vi "Main.vi"(10 "Coins Panel":refnum<vi>, 11 "Module Admin":refnum<class "Delacor_lib_QMH_Module Admin.lvclass">) -> ()   [LabVIEW 2019, in "COINS.lvlib"]
doc: "This template is based off of the Queued Message Handler design pattern and the Queued Message Handler project template that ships with LabVIEW.\n\nThe main difference is that the queue is private to this module and communication between modules is performed via Broadcast and Request events.\n\nRequest events are wrapped in public API methods and are handled in the Event Handling Loop (EHL) of this VI. Any module can register for Broadcast events sent by this module. The EHL generates messages based on user interface actions.\n\nThe Message Handling Loop (MHL) processes messages generated by the EHL, or by other messages. The messages are string values, so new messages can be added easily to the Message Cases case structure in the MHL. Each message cluster can also provide an optional value for Message Data, which is a variant that can be converted to whatever message-specific data is required.\n_____\nBased on Delacor QMH Project Template 5.0.0.82."
uses:
  COINS.lvlib
  <vilib>/Delacor/Delacor QMH/Libraries/Module Admin_class/Delacor_lib_QMH_Module Admin.lvclass
  Module Data--cluster.ctl
  Stop Argument--cluster.ctl
  <vilib>/Delacor/Delacor QMH/Libraries/Message Queue_class/Delacor_lib_QMH_Message Queue.lvclass/Delacor_lib_QMH_Message Queue.ctl
  <vilib>/Delacor/Delacor QMH/Libraries/Module Admin_class/Delacor_lib_QMH_Module Admin.lvclass/Delacor_lib_QMH_Module Admin.ctl
  SET COINS Argument--cluster.ctl
  UPDATE COIN Argument--cluster.ctl
  UPDATE CREDIT Argument--cluster.ctl
  <vilib>/Delacor/Delacor QMH/Libraries/Message Queue_class/Delacor_lib_QMH_Enqueue Message (Single).vi
  <vilib>/Delacor/Delacor QMH/Libraries/Module Admin_class/Delacor_lib_QMH_Get External Launch.vi
  <vilib>/Utility/error.llb/Error Cluster From Error Code.vi
  <vilib>/ErrorRing/Error Ring.xnode
  <vilib>/Delacor/Delacor QMH/Libraries/Message Queue_class/Delacor_lib_QMH_Message Queue.lvclass
  MESSAGES/MESSAGES.lvlib
panel:
  in  "COIN 1":bool
  in  "COIN 2":bool
  in  "COIN 3":bool
  in  "COIN 4":bool
  out "error out":errorcluster
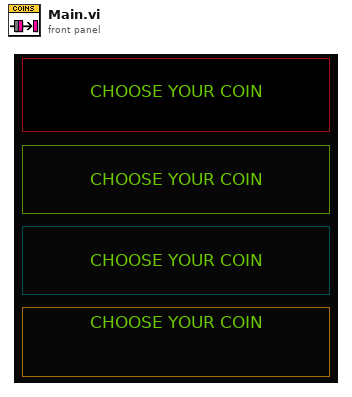
[diagram p1: front panel]
types:
  T1 = typedef "COINS.lvlib/Request Events--cluster.ctl" = cluster{"Stop Module":refnum<user-event>, "Show Panel":refnum<user-event>, "Hide Panel":refnum<user-event>, "Get Module Execution Status":refnum<user-event>, "Show Diagram":refnum<user-event>, "SET COINS":refnum<user-event>, "UPDATE COIN":refnum<user-event>, "UPDATE CREDIT":refnum<user-event>}
  T2 = typedef "COINS.lvlib/Module Data--cluster.ctl" = cluster{"Status":string, "CREDIT":dbl, "PRICE":dbl, "CHANGE":dbl, "MONEY COINS":string[], "MONEY VALUES":string[], "COINS":bool[]}
  T3 = enum32{"invalid lock state", "Not Locked", "Locked (No Password)", "Password-protected"}
  T4 = typedef "COINS.lvlib/Stop Argument--cluster.ctl" = cluster{"Origin":string, "Exit via Stop Module Req?":bool, "Wait for Module to stop?":bool}
  T5 = typedef "COINS.lvlib/SET COINS Argument--cluster.ctl" = cluster{"MONEY ARRAY":string[]}
  T6 = typedef "COINS.lvlib/UPDATE COIN Argument--cluster.ctl" = cluster{"Boolean":bool}
  T7 = typedef "COINS.lvlib/UPDATE CREDIT Argument--cluster.ctl" = cluster{"Boolean":bool}
  T8 = enum32{"Invalid", "Standard", "Closed", "Hidden", "Minimized", "Maximized"}
  T9 = cluster{"MONEY ARRAY[0]":string, "MONEY ARRAY[1]":string, "MONEY ARRAY[2]":string, "MONEY ARRAY[3]":string, "MONEY ARRAY[4]":string, "MONEY ARRAY[5]":string, "MONEY ARRAY[6]":string, "MONEY ARRAY[7]":string, "MONEY ARRAY[8]":string}
  T10 = cluster{"MONEY COINS[0]":string, "MONEY COINS[1]":string, "MONEY COINS[2]":string, "MONEY COINS[3]":string, "MONEY COINS[4]":string, "MONEY COINS[5]":string, "MONEY COINS[6]":string, "MONEY COINS[7]":string, "MONEY COINS[8]":string}
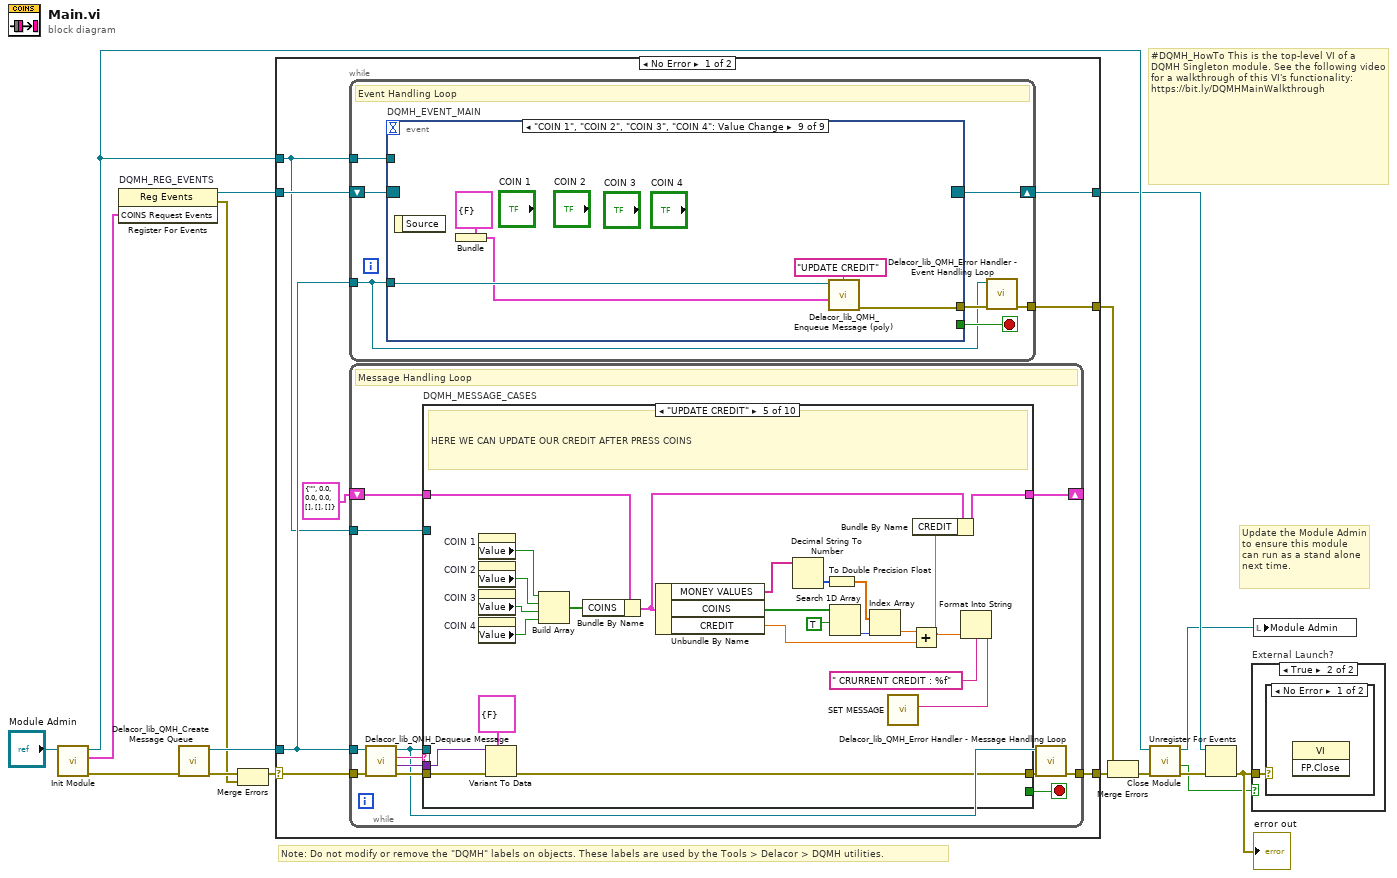
[diagram p0: block diagram]
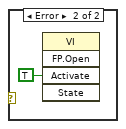
[diagram p3: hidden frame]
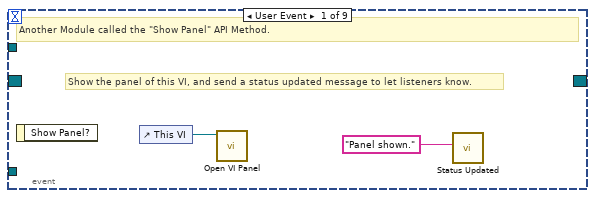
[diagram p4: hidden frame]
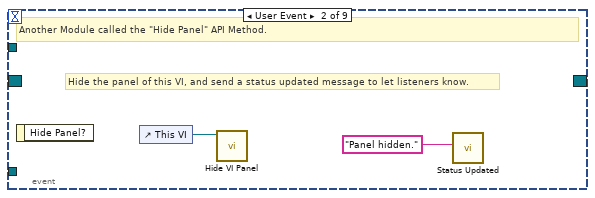
[diagram p5: hidden frame]
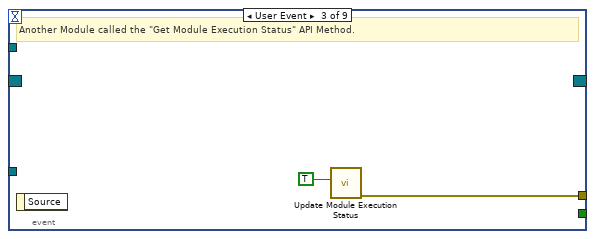
[diagram p6: hidden frame]
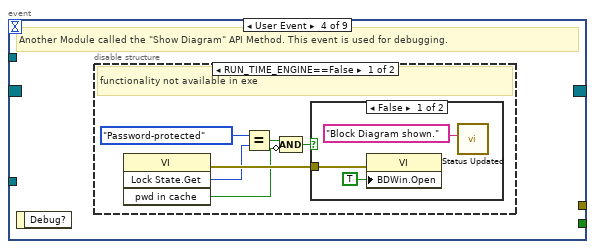
[diagram p7: hidden frame]
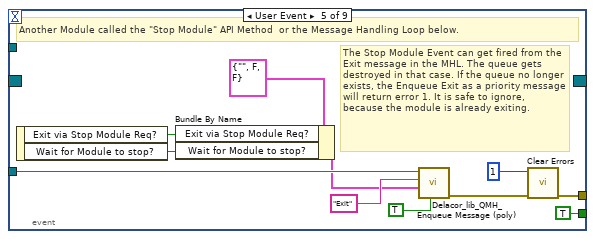
[diagram p10: hidden frame]
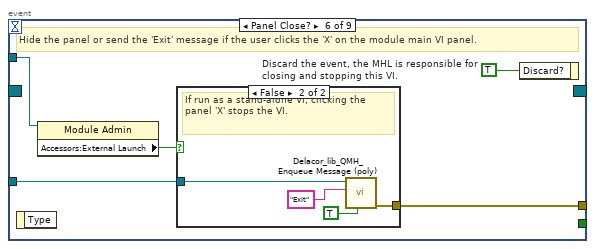
[diagram p11: hidden frame]
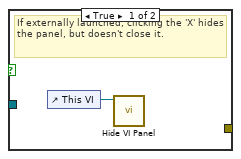
[diagram p12: hidden frame]
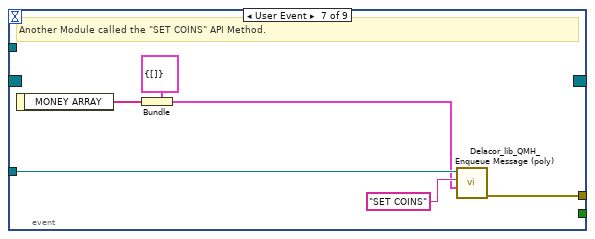
[diagram p13: hidden frame]
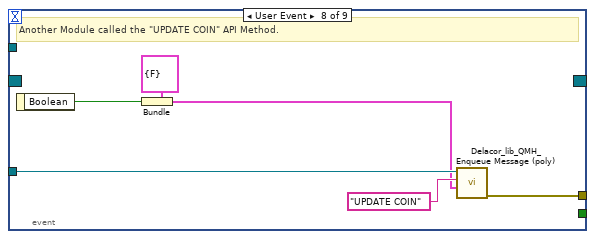
[diagram p14: hidden frame]
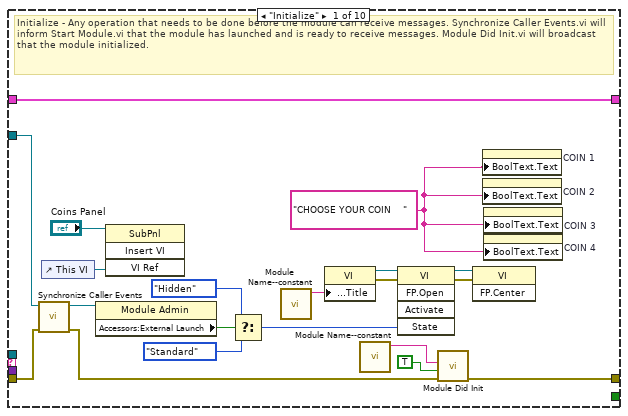
[diagram p15: hidden frame]
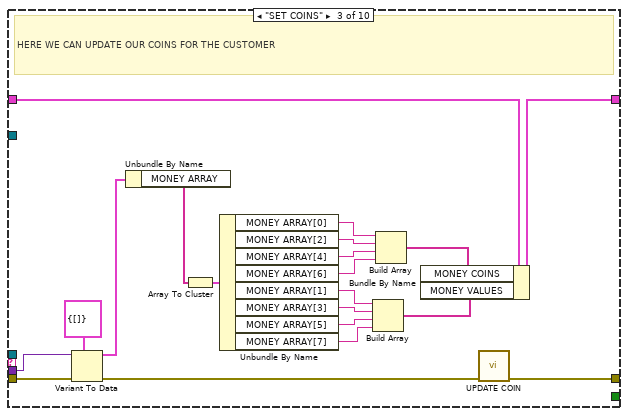
[diagram p17: hidden frame]
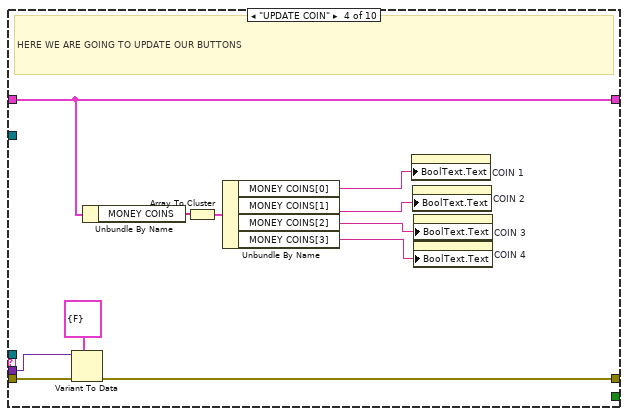
[diagram p18: hidden frame]
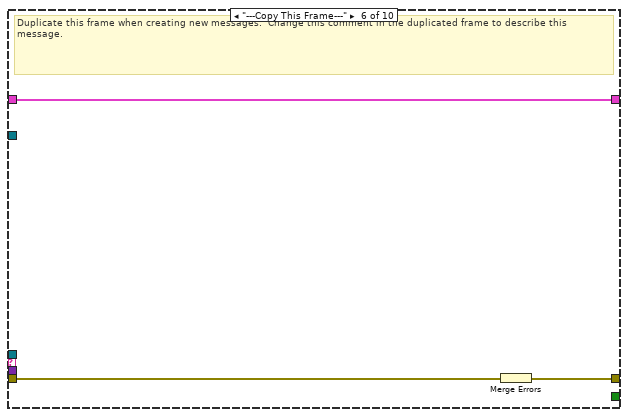
[diagram p19: hidden frame]
diagram:
  # "#DQMH_HowTo This is the top-level VI of a DQMH Singleton module. See the following video for a walkthrough of this VI's functionality: https://bit.ly/DQMHMainWalkthrough"
  # "Note: Do not modify or remove the \"DQMH\" labels on objects. These labels are used by the Tools > Delacor > DQMH utilities."
  # "Update the Module Admin to ensure this module can run as a stand alone next time."
  n1 = call "Init Module.vi"("Singleton Module Admin in"="Module Admin") -> ("error out"=w16:errorcluster, "COINS Request Events"=w6:T1, "Singleton Module Admin out"=w9:refnum<class "Delacor_lib_QMH_Module Admin.lvclass">)  [unwired: 8 in]
  n2 = register-events "DQMH_REG_EVENTS"(w6) -> (reference out=w7:refnum<event-registration>, error out=w1:errorcluster)  [unwired: 2 in]
  n3 = call <vilib>:"Delacor_lib_QMH_Create Message Queue.vi"("error in (no error)"=w16) -> ("error out"=w11:errorcluster, "Message Queue"=w5:refnum<class "Delacor_lib_QMH_Message Queue.lvclass">)  [unwired: 9 in]
  n4 = Merge Errors(w11, w1) -> (w10:errorcluster)
  n5 = case shown="No Error" w10 {
    selector: w10 -> [w23 w227]
    tunnel: [w25 w226] -> w17
    tunnel: [w22 w232] -> w8
    tunnel: w7 -> [w20 w232]
    tunnel: w5 -> [w19 w225]
    tunnel: [w24 _] -> w14
    tunnel: w9 -> [w18 w228]
    frame No Error {
      n6 = while {
        tunnel: w19 -> [w26]
        shift-right: [w29] -> w22
        shift-left: w20 -> [w30]
        tunnel: [w31] -> w24
        tunnel: w18 -> [w27]
        stop <- w28 stop-if-true
        # "Event Handling Loop"
        n7 = event "DQMH_EVENT_MAIN" shown="[8] \"COIN 1\", \"COIN 2\", \"COIN 3\", \"COIN 4\": Value Change" {
          selector: w30 -> [_ _ _ _ _ _ _ _ _]
          dyn-events: [_ _ _ _ _ _ _ _ _] -> w29
          timeout: _ -> [_ _ _ _ _ _ _ _ _]
          tunnel: [_ _ _ _ TRUE ("Discard?") _ _ _ _] -> w28
          tunnel: w26 -> [_ _ _ _ w54 w61 w74 w80 w83]
          tunnel: [_ _ w38 _ w57 w63 w69 w75 w84] -> w32
          tunnel: w27 -> [_ _ _ _ _ w60 _ _ _]
          event User Event {
            # "Show the panel of this VI, and send a status updated message to let listeners know."
            # "Another Module called the \"Show Panel\" API Method."
            n8 = event-data() -> ()  [unwired: 1 in, 1 out]
            n9 = control-ref of="This VI"() -> (w34:refnum<vi>)
            n10 = call "Open VI Panel.vi"("VI"=w34) -> ()  [unwired: 10 in, 1 out]
            n11 = call "Status Updated.vi"("Status"="Panel shown." ("format string")) -> ()  [unwired: 10 in, 1 out]
          }
          event User Event {
            # "Hide the panel of this VI, and send a status updated message to let listeners know."
            # "Another Module called the \"Hide Panel\" API Method."
            n12 = event-data() -> ()  [unwired: 1 in, 1 out]
            n13 = control-ref of="This VI"() -> (w36:refnum<vi>)
            n14 = call "Hide VI Panel.vi"("VI"=w36) -> ()  [unwired: 10 in, 1 out]
            n15 = call "Status Updated.vi"("Status"="Panel hidden." ("format string")) -> ()  [unwired: 10 in, 1 out]
          }
          event User Event {
            # "Another Module called the \"Get Module Execution Status\" API Method."
            n16 = event-data() -> ()  [unwired: 1 in, 1 out]
            n17 = call "Update Module Execution Status.vi"("Running?"=TRUE) -> ("error out"=w38:errorcluster)  [unwired: 10 in]
          }
          event User Event {
            # "Another Module called the \"Show Diagram\" API Method. This event is used for debugging."
            n18 = event-data() -> ()  [unwired: 1 in, 1 out]
            n19 = disable-structure shown="RUN_TIME_ENGINE==False" {
              frame condition #0 (active) {
                # "functionality not available in exe"
                n20 = invoke class="VI" method="Lock State.Get"() -> (error out=w44:errorcluster, "Get Lock State"=w43:T3, "pwd in cache"=w40:bool)  [unwired: 4 in, 1 out]
                n21 = Equal?(x=T3."Password-protected", y=w43) -> (x = y?=w41:bool)
                n22 = Compound Arithmetic op=AND(w41, invert w40) -> (w39:bool)
                n23 = case shown="False" w39 {
                  tunnel: w44 -> [w47 _]
                  frame False {
                    n24 = property class="VI"(error in=w47, "BDWin.Open"=TRUE ("Block Diagram Window:Open")) -> ()  [unwired: 1 in, 2 out]
                    n25 = call "Status Updated.vi"("Status"="Block Diagram shown." ("format string")) -> ()  [unwired: 10 in, 1 out]
                  }
                  frame True {
                    # "Password-protected VI, and the password is not in the cache. Do not show the diagram."
                  }
                }
              }
              frame condition #1 {
              }
            }
          }
          event User Event {
            # "The Stop Module Event can get fired from the Exit message in the MHL. The queue gets destroyed in that case. If the queue no longer exists, the Enqueue Exit as a priority message will return error 1. It is safe to ignore, because the module is already exiting."
            # "Another Module called the \"Stop Module\" API Method  or the Message Handling Loop below."
            n26 = event-data() -> ("Exit via Stop Module Req?"=w50:bool, "Wait for Module to stop?"=w49:bool)  [unwired: 1 in]
            n27 = Bundle By Name(cluster=T4 {"Origin"="", "Exit via Stop Module Req?"=FALSE, "Wait for Module to stop?"=FALSE} ("Stop Argument"), "Exit via Stop Module Req?"=w50, "Wait for Module to stop?"=w49) -> (w48:T4)
            n28 = call-poly <vilib>:"Delacor_lib_QMH_Enqueue Message (poly).vi"("Priority Message? (F)"=TRUE, "Message Data"=w48, "Message"="Exit", "Message Queue in"=w54) -> ("error out"=w58:errorcluster)  [unwired: 6 in, 1 out]
            n29 = call <vilib>:"Clear Errors.vi"("error in (no error)"=w58, "specific error code to clear (0: all)"=1) -> ("error out"=w57:errorcluster)  [unwired: 4 in, 1 out]
          }
          event Panel Close? {
            w62 = TRUE  # Discard the event, the MHL is responsible for closing and stopping this VI.
            # "Hide the panel or send the 'Exit' message if the user clicks the 'X' on the module main VI panel."
            n30 = event-data() -> ()  [unwired: 1 in, 1 out]
            n31 = property class="Module Admin"(reference=w60) -> ("Accessors:External Launch"=w59:bool)  [unwired: 1 in, 2 out]
            n32 = case shown="False" w59 {
              tunnel: w61 -> [_ w67]
              tunnel: [_ w68] -> w63
              frame True {
                # "If externally launched, clicking the 'X' hides the panel, but doesn't close it."
                n33 = control-ref of="This VI"() -> (w64:refnum<vi>)
                n34 = call "Hide VI Panel.vi"("VI"=w64) -> ()  [unwired: 10 in, 1 out]
              }
              frame False {
                # "If run as a stand-alone VI, clicking the panel 'X' stops the VI."
                n35 = call-poly <vilib>:"Delacor_lib_QMH_Enqueue Message (poly).vi"("Priority Message? (F)"=TRUE, "Message"="Exit", "Message Queue in"=w67) -> ("error out"=w68:errorcluster)  [unwired: 7 in, 1 out]
              }
            }
            n36 = event-data("Discard?"=w62) -> ()  [unwired: 1 in, 1 out]
          }
          event User Event {
            # "Another Module called the \"SET COINS\" API Method."
            n37 = event-data() -> ("MONEY ARRAY"=w70:string[])  [unwired: 1 in]
            n38 = Bundle(cluster=T5 {"MONEY ARRAY"=[]} ("SET COINS Argument"), "MONEY ARRAY"=w70) -> (w71:T5)
            n39 = call-poly <vilib>:"Delacor_lib_QMH_Enqueue Message (poly).vi"("Message Data"=w71, "Message"="SET COINS", "Message Queue in"=w74) -> ("error out"=w69:errorcluster)  [unwired: 7 in, 1 out]
          }
          event User Event {
            # "Another Module called the \"UPDATE COIN\" API Method."
            n40 = event-data() -> ("Boolean"=w76:bool)  [unwired: 1 in]
            n41 = Bundle(cluster=T6 {"Boolean"=FALSE} ("UPDATE COIN Argument"), "Boolean"=w76) -> (w77:T6)
            n42 = call-poly <vilib>:"Delacor_lib_QMH_Enqueue Message (poly).vi"("Message Data"=w77, "Message"="UPDATE COIN", "Message Queue in"=w80) -> ("error out"=w75:errorcluster)  [unwired: 7 in, 1 out]
          }
          event "COIN 1", "COIN 2", "COIN 3", "COIN 4": Value Change {
            n43 = event-data() -> ()  [unwired: 1 in, 1 out]
            n44 = Bundle(cluster=T7 {"Boolean"=FALSE} ("UPDATE CREDIT Argument")) -> (w81:T7)  [unwired: 1 in]
            n45 = call-poly <vilib>:"Delacor_lib_QMH_Enqueue Message (poly).vi"("Message Data"=w81, "Message"="UPDATE CREDIT", "Message Queue in"=w83) -> ("error out"=w84:errorcluster)  [unwired: 7 in, 1 out]
          }
        }
        n46 = call-dynamic "Delacor_lib_QMH_Error Handler - Event Handling Loop.vi"("error in (no error)"=w32, "Message Queue in"=w26) -> ("dup error in"=w31:errorcluster)  [unwired: 8 in, 1 out]
      }
      n47 = while {
        tunnel: w19 -> [w88]
        shift-right: [w92] -> _
        shift-left: T2 {"Status"="", "CREDIT"=0.0, "PRICE"=0.0, "CHANGE"=0.0, "MONEY COINS"=[], "MONEY VALUES"=[], "COINS"=[]} ("Data Cluster") -> [w93]
        tunnel: w23 -> [w96]
        tunnel: [w94] -> w25
        tunnel: w18 -> [w86]
        stop <- w91 stop-if-true
        # "Message Handling Loop"
        n48 = call-dynamic "Delacor_lib_QMH_Dequeue Message.vi"("error in (no error)"=w96, "Message Queue in"=w88) -> ("error out"=w95:errorcluster, "Message Data"=w89:variant, "Message"=w90:string, "Message Queue out"=w87:refnum<class "Delacor_lib_QMH_Message Queue.lvclass">)  [unwired: 6 in]
        n49 = case "DQMH_MESSAGE_CASES" shown="\"UPDATE CREDIT\"" w90 {
          selector: w90 -> [_ _ _ _ _ _ _ _ _ w212]
          tunnel: w87 -> [_ _ _ _ _ _ _ w182 w204 _]
          tunnel: w95 -> [w115 w119 w139 w150 w173 w176 w178 w189 w210 w214]
          tunnel: [w100 w119 w120 w149 w172 w175 w178 w185 w207 w215] -> w97
          tunnel: w93 -> [w98 w118 w138 w141 w157 w174 w177 w184 w203 w213]
          tunnel: [w98 w118 w132 w141 w159 w174 w177 w184 w203 w213] -> w92
          tunnel: [_ _ _ _ _ _ _ _ w202 _] -> w91
          tunnel: w89 -> [_ _ w137 w148 w171 _ _ w183 w201 _]
          tunnel: w86 -> [w106 _ _ _ _ _ _ w181 w196 _]
          frame "Initialize" {
            w99 = "CHOOSE YOUR COIN    "
            # "Initialize - Any operation that needs to be done before the module can receive messages. Synchronize Caller Events.vi will inform Start Module.vi that the module has launched and is ready to receive messages. Module Did Init.vi will broadcast that the module initialized."
            n50 = call "Synchronize Caller Events.vi"("error in (no error)"=w115, "Singleton Module Admin in"=w106) -> ("error out"=w114:errorcluster, "Singleton Module Admin out"=w103:refnum<class "Delacor_lib_QMH_Module Admin.lvclass">)  [unwired: 8 in]
            n51 = control-ref of="This VI"() -> (w102:refnum<vi>)
            n52 = property class="Module Admin"(reference=w103) -> ("Accessors:External Launch"=w110:bool)  [unwired: 1 in, 2 out]
            n53 = invoke class="SubPnl" method="Insert VI"(reference="Coins Panel", "VI Ref"=w102) -> ()  [unwired: 2 in, 4 out]
            n54 = Select(t=T8."Hidden" ("State"), s=w110, f=T8."Standard" ("State")) -> (s? t:f=w107:T8)
            n55 = call "Module Name--constant.vi"() -> ("Module Name"=w113:string)  [unwired: 11 in]
            n56 = property class="VI"("Front Panel.Title"=w113) -> (reference out=w112:refnum<vi>, error out=w117:errorcluster)  [unwired: 2 in]
            n57 = call "Module Name--constant.vi"() -> ("Module Name"=w104:string)  [unwired: 11 in]
            n58 = invoke class="VI" method="FP.Open"(reference=w112, error in=w117, "State"=w107) -> (reference out=w111:refnum<vi>, error out=w116:errorcluster)  [unwired: 2 in, 3 out]
            n59 = call "Module Did Init.vi"("error in (no error)"=w114, "Initialized?"=TRUE, "Origin"=w104) -> ("error out"=w100:errorcluster)  [unwired: 8 in]
            n60 = invoke class="VI" method="FP.Center"(reference=w111, error in=w116) -> ()  [unwired: 1 in, 3 out]
            n61 = property on="COIN 1" class="Bool (strict)"("BoolText.Text"=w99) -> ()  [unwired: 2 in, 2 out]
            n62 = property on="COIN 2" class="Bool (strict)"("BoolText.Text"=w99) -> ()  [unwired: 2 in, 2 out]
            n63 = property on="COIN 3" class="Bool (strict)"("BoolText.Text"=w99) -> ()  [unwired: 2 in, 2 out]
            n64 = property on="COIN 4" class="Bool (strict)"("BoolText.Text"=w99) -> ()  [unwired: 2 in, 2 out]
          }
          frame "--- Module Specific ---" {
            # "Separator -- The following cases handle messages specific to this Module."
          }
          frame "SET COINS" {
            # "HERE WE CAN UPDATE OUR COINS FOR THE CUSTOMER"
            n65 = Variant To Data(error in=w139, type=T5 {"MONEY ARRAY"=[]} ("SET COINS Argument"), Variant=w137) -> (data=w135:T5, error out=w121:errorcluster)
            n66 = Unbundle By Name(w135) -> ("MONEY ARRAY"=w133:string[])
            n67 = Array To Cluster(array=w133) -> (cluster=w134:T9)
            n68 = Unbundle By Name(w134) -> ("MONEY ARRAY[0]"=w131:string, "MONEY ARRAY[2]"=w130:string, "MONEY ARRAY[4]"=w129:string, "MONEY ARRAY[6]"=w128:string, "MONEY ARRAY[1]"=w126:string, "MONEY ARRAY[3]"=w125:string, "MONEY ARRAY[5]"=w124:string, "MONEY ARRAY[7]"=w123:string)
            n69 = Build Array(w126, w125, w124, w123) -> (w122:string[])
            n70 = Build Array(w131, w130, w129, w128) -> (w127:string[])
            n71 = Bundle By Name(cluster=w138, "MONEY COINS"=w127, "MONEY VALUES"=w122) -> (w132:T2)
            n72 = call "UPDATE COIN.vi"("error in (no error)"=w121) -> ("error out"=w120:errorcluster)  [unwired: 10 in]
          }
          frame "UPDATE COIN" {
            # "HERE WE ARE GOING TO UPDATE OUR BUTTONS"
            n73 = Variant To Data(error in=w150, type=T6 {"Boolean"=FALSE} ("UPDATE COIN Argument"), Variant=w148) -> (error out=w149:errorcluster)  [unwired: 1 out]
            n74 = Unbundle By Name(w141) -> ("MONEY COINS"=w142:string[])
            n75 = Array To Cluster(array=w142) -> (cluster=w146:T10)
            n76 = Unbundle By Name(w146) -> ("MONEY COINS[0]"=w140:string, "MONEY COINS[1]"=w145:string, "MONEY COINS[2]"=w144:string, "MONEY COINS[3]"=w143:string)
            n77 = property on="COIN 1" class="Bool (strict)"("BoolText.Text"=w140) -> ()  [unwired: 2 in, 2 out]
            n78 = property on="COIN 2" class="Bool (strict)"("BoolText.Text"=w145) -> ()  [unwired: 2 in, 2 out]
            n79 = property on="COIN 3" class="Bool (strict)"("BoolText.Text"=w144) -> ()  [unwired: 2 in, 2 out]
            n80 = property on="COIN 4" class="Bool (strict)"("BoolText.Text"=w143) -> ()  [unwired: 2 in, 2 out]
          }
          frame "UPDATE CREDIT" {
            # "HERE WE CAN UPDATE OUR CREDIT AFTER PRESS COINS"
            n81 = property on="COIN 1" class="Bool (strict)"() -> ("Value"=w155:bool)  [unwired: 2 in, 2 out]
            n82 = property on="COIN 2" class="Bool (strict)"() -> ("Value"=w154:bool)  [unwired: 2 in, 2 out]
            n83 = property on="COIN 3" class="Bool (strict)"() -> ("Value"=w153:bool)  [unwired: 2 in, 2 out]
            n84 = property on="COIN 4" class="Bool (strict)"() -> ("Value"=w152:bool)  [unwired: 2 in, 2 out]
            n85 = Variant To Data(error in=w173, type=T7 {"Boolean"=FALSE} ("UPDATE CREDIT Argument"), Variant=w171) -> (error out=w172:errorcluster)  [unwired: 1 out]
            n86 = Build Array(w155, w154, w153, w152) -> (w151:bool[])
            n87 = Bundle By Name(cluster=w157, "COINS"=w151) -> (w156:T2)
            n88 = Unbundle By Name(w156) -> ("MONEY VALUES"=w167:string[], "COINS"=w158:bool[], "CREDIT"=w160:dbl)
            n89 = Decimal String To Number(string=w167) -> (number=w166:i32[])  [unwired: 2 in, 1 out]
            n90 = To Double Precision Float(number=w166) -> (double precision float=w165:dbl[])
            n91 = Search 1D Array(1D array=w158, element=TRUE) -> (index of element=w168:i32)  [unwired: 1 in]
            n92 = Index Array(array=w165, index=w168) -> (element=w164:dbl)
            n93 = Add(x=w164, y=w160) -> (x+y=w162:dbl)
            n94 = Bundle By Name(cluster=w156, "CREDIT"=w162) -> (w159:T2)
            n95 = Format Into String(format string=" CRURRENT CREDIT : %f", w162) -> (resulting string=w161:string)  [unwired: 2 in, 1 out]
            n96 = call "SET MESSAGE.vi"("Message"=w161) -> ()  [unwired: 10 in, 1 out]
          }
          frame "---Copy This Frame---" {
            # "Duplicate this frame when creating new messages.  Change this comment in the duplicated frame to describe this message."
            n97 = Merge Errors(w176) -> (w175:errorcluster)
          }
          frame "--- Exit and Error Handling---" {
            # "Separator - The following cases handle errors and exit messages."
          }
          frame "Error" {
            # "#CodeRecommended - If you ever change the name of this \"Error\" message, you'll need to update the name in the Check Loop Error.vi as well."
            # "#CodeRecommended - If the module is running in standalone mode (External Launch = FALSE), this code will pop up an error dialog and call the 'Exit' message if an error occurs. Add more fine-grained error handling here."
            # "Error - Check the error message data and respond accordingly. This message is sent by the \"Error Handler\" VIs at the end of each loop in this application."
            n98 = property class="Module Admin"(reference=w181) -> ("Accessors:External Launch"=w180:bool)  [unwired: 1 in, 2 out]
            n99 = Variant To Data(error in=w189, type=errorcluster {"status"=FALSE, "code"=0, "source"=""} ("error constant"), Variant=w183) -> (data=w190:errorcluster, error out=w187:errorcluster)
            n100 = call "Module Name--constant.vi"() -> ("Module Name"=w179:string)  [unwired: 11 in]
            n101 = call "Error Reported.vi"("Additional Information"=w179, "Error"=w190) -> ()  [unwired: 9 in, 1 out]
            n102 = case shown="False" w180 {
              tunnel: [w195 _] -> w186
              tunnel: w182 -> [w193 _]
              tunnel: w190 -> [w194 _]
              frame False {
                # "If the module is running standalone, then pop up an error dialog and call the \"Exit\" message."
                n103 = call <vilib>:"Simple Error Handler.vi"("error in (no error)"=w194) -> ()  [unwired: 4 in, 5 out]
                n104 = call-poly <vilib>:"Delacor_lib_QMH_Enqueue Message (poly).vi"("Priority Message? (F)"=TRUE, "Message"="Exit", "Message Queue in"=w193) -> ("error out"=w195:errorcluster)  [unwired: 7 in, 1 out]
              }
              frame True {
                # "If the module was launched externally, calling the Error Reported broadcast VI is the only action performed by the \"Error\" message. The module's caller can then process the error appropriately."
              }
            }
            n105 = Merge Errors(w187, w186) -> (w185:errorcluster)
            n106 = local write "error out"(w185) -> ()
          }
          frame "Exit" {
            w200 = 91  # 91: not all Exit messages will have an argument
            w202 = TRUE  # Stop the VI
            # "Release the message queue reference"
            # "#CodeNeeded - Add any required cleanup code here"
            # "Exit - Exit the application."
            n107 = Variant To Data(error in=w210, type=T4 {"Origin"="", "Exit via Stop Module Req?"=FALSE, "Wait for Module to stop?"=FALSE} ("Stop Argument"), Variant=w201) -> (data=w198:T4, error out=w206:errorcluster)
            n108 = call <vilib>:"Clear Errors.vi"("error in (no error)"=w206, "specific error code to clear (0: all)"=w200) -> ("error out"=w209:errorcluster)  [unwired: 4 in, 1 out]
            n109 = control-ref of="This VI"() -> (w197:refnum<vi>)
            n110 = call-dynamic "Delacor_lib_QMH_Release Message Queue.vi"("error in (no error)"=w209, "Message Queue"=w204) -> ("error out"=w208:errorcluster)  [unwired: 9 in]
            n111 = call "Handle Exit.vi"("Stop Argument"=w198, "Admin in"=w196, "VI reference"=w197) -> ("error out"=w205:errorcluster)  [unwired: 7 in, 1 out]
            n112 = Merge Errors(w208, w205) -> (w207:errorcluster)
          }
          frame Default {
            # "'Default' case only runs if there is a message that isn't defined in any of the other cases.  Output a programming error."
            n113 = call "Module Name--constant.vi"() -> ("Module Name"=w211:string)  [unwired: 11 in]
            n114 = xnode "Error Ring"("parameter 0"=w212, "parameter 1"=w211) -> ("error out"=w216:errorcluster)
            n115 = Merge Errors(w214, w216) -> (w215:errorcluster)
          }
        }
        n116 = call-dynamic "Delacor_lib_QMH_Error Handler - Message Handling Loop.vi"("error in (no error)"=w97, "Message Queue in"=w87) -> ("dup error in"=w94:errorcluster)  [unwired: 8 in, 1 out]
      }
    }
    frame Error {
      # "Synchronize Caller Events.vi will inform Start Module.vi that the module has launched and will let the code calling Start Module.vi register for broadcasts and would permit the caller receive the broadcast that an error occurred at launch time."
      n117 = call-dynamic "Delacor_lib_QMH_Release Message Queue.vi"("error in (no error)"=w227, "Message Queue"=w225) -> ("error out"=w226:errorcluster)  [unwired: 9 in]
      n118 = call "Synchronize Caller Events.vi"("Singleton Module Admin in"=w228) -> ("error out"=w233:errorcluster)  [unwired: 9 in, 1 out]
      n119 = call "Module Name--constant.vi"() -> ("Module Name"=w231:string)  [unwired: 11 in]
      n120 = Format Into String(format string="An error occurred during initialization. %s is no longer running.", w231) -> (resulting string=w229:string)  [unwired: 2 in, 1 out]
      n121 = Merge Errors(w226, w233) -> (w234:errorcluster)
      n122 = call "Error Reported.vi"("Additional Information"=w229, "Error"=w234) -> ()  [unwired: 9 in, 1 out]
    }
  }
  n123 = Merge Errors(w14, w17) -> (w13:errorcluster)
  n124 = call "Close Module.vi"("error in (no error)"=w13, "Module Admin in"=w9) -> ("error out"=w15:errorcluster, "External Launch"=w2:bool, "Module Admin out"=w3:refnum<class "Delacor_lib_QMH_Module Admin.lvclass">)  [unwired: 7 in]
  n125 = Unregister For Events(event registration refnum=w8, error in=w15) -> (error out=w12:errorcluster)
  "error out" <- w12
  n126 = case "External Launch?" shown="True" w2 {
    tunnel: w12 -> [_ w235]
    frame False {
    }
    frame True {
      n127 = case shown="No Error" w235 {
        frame No Error {
          n128 = invoke class="VI" method="FP.Close"() -> ()  [unwired: 3 in, 3 out]
        }
        frame Error {
          n129 = invoke class="VI" method="FP.Open"("Activate"=TRUE ("Activate?")) -> ()  [unwired: 4 in, 5 out]
        }
      }
    }
  }
  n130 = local write "Module Admin"(w3) -> ()
